vi "Teleop.vi"(10 "Match Info":T3={"Autonomous Elapsed Seconds"=0.0, "TeleOp Elapsed Seconds"=0.0, "Disabled Elapsed Seconds"=0.0, "Visited Autonomous"=FALSE, "Visited TeleOp"=FALSE, "Visited Disabled"=FALSE, "Autonomous Settings"={"Autonomous Style"=enum."Independent", "VI Refnum"=refnum}}, 11 "Call Context":T4) -> ()   [LabVIEW 2020]
doc: "This VI is called for each TeleOp packet received from the DS where the robot is not disabled. It is often used to read from the joysticks and update I/O or to update setpoints for timed control loops. It should complete and return within 20 milliseconds or it may miss DS packets."
uses:
  <vilib>/Rock Robotics/WPI/DriverStation/WPI_DriverStationDerivedRobotMode.ctl
  <vilib>/Rock Robotics/WPI/DriverStation/WPI_DriverStationMatch Info.ctl
  <vilib>/Rock Robotics/WPI/ThirdParty/Sensors/navX/_TypeDefs/FRIC_navX_DeviceNumbersTypeDef.ctl
  981LabViewComponents/2023 Robot Global Data.vi
  <vilib>/Rock Robotics/WPI/Utilities/WPI_GetSetVariantRefNum.vi
  <vilib>/Rock Robotics/Network Tables/NT Write Boolean Array.vi
  <vilib>/Rock Robotics/Network Tables/NT Write Numeric Array.vi
  <vilib>/Rock Robotics/Network Tables/NT Read Boolean.vi
  <vilib>/Rock Robotics/Network Tables/NT Read Number.vi
  <vilib>/Rock Robotics/Network Tables/NT Write Number.vi
panel:
  out "armSensor":dbl
  out "wristSensor":dbl
  out "armTarget":dbl
  out "wristTarget":dbl
  out "teleopState":T1(ring)
  out "displayTeleopCounter":i32
  out "Raw Values":T2 {"Accel X" format="%.8f"; "Accel Y" format="%.8f"; "Accel Z" format="%.8f"; "Gyro X" format="%.8f"; "Gyro Y" format="%.8f"; "Gyro Z" format="%.8f"; "Mag X" format="%.8f"; "Mag Y" format="%.8f"; "Mag Z" format="%.8f"}
  out "Sample Slider 0":dbl(slide) scale=0.0..5.0
  out "Sample Boolean 1":bool
  out "Sample Boolean 0":bool
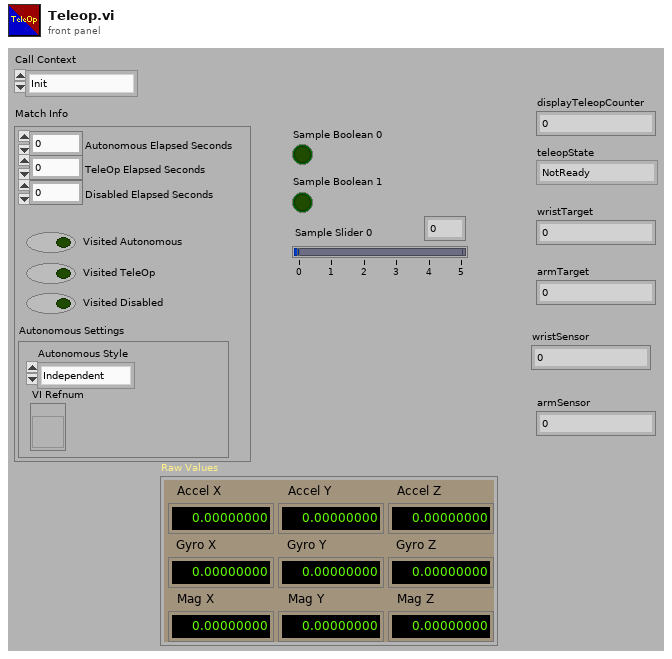
[diagram p1: front panel]
types:
  T1 = enum16{"NotReady", "Init", "UnstowA", "UnstowB", "UnstowC", "Teleop", "StowA", "StowB", "StowC"}
  T2 = cluster{"Accel X":dbl, "Accel Y":dbl, "Accel Z":dbl, "Gyro X":dbl, "Gyro Y":dbl, "Gyro Z":dbl, "Mag X":dbl, "Mag Y":dbl, "Mag Z":dbl}
  T3 = typedef "WPI_DriverStationMatch Info.ctl" = cluster{"Autonomous Elapsed Seconds":dbl, "TeleOp Elapsed Seconds":dbl, "Disabled Elapsed Seconds":dbl, "Visited Autonomous":bool, "Visited TeleOp":bool, "Visited Disabled":bool, "Autonomous Settings":cluster{"Autonomous Style":enum16{"Iterative", "Independent"}, "VI Refnum":refnum<vi>}}
  T4 = typedef "WPI_DriverStationDerivedRobotMode.ctl" = enum16{"Init", "Execute", "Stop"}
  T5 = typedef "WPI_JoystickDevRef.ctl" = cluster{"Device":T6}
  T6 = typedef "WPI_JoystickDeviceEnum.ctl" = enum16{"USB 0", "USB 1", "USB 2", "USB 3", "USB 4", "USB 5"}
  T7 = typedef "FRIC_navX_DeviceNumbersTypeDef.ctl" = enum16{"Dev0", "Dev1", "Dev2", "Dev3"}
  T8 = typedef "WPI_RobotDriveDevRef.ctl" = cluster{"DevStatus":errorcluster, "Motors[]":T9[], "Square Inputs":bool, "Max Output":dbl}
  T9 = typedef "WPI_MotorControlDeviceRef.ctl" = cluster{"DeviceStatus":errorcluster, "Type":T10, "PWM":cluster{"PWM Channel":T11, "DeadBand":T12}, "CAN":cluster{"Device Number":u8, "SetOutput VI Ref":variant, "GetOutput VI Ref":variant, "Enable VI Ref":variant, "Disable VI Ref":variant, "Data":variant}, "Invert":bool, "DIO PWM":cluster{"PWM \"Enable\" Channel":T11, "DIOChannel":T13, "PWM Rate":dbl}}
  T10 = typedef "WPI_MotorControlType.ctl" = enum16{"PWM", "CAN", "DIO PWM"}
  T11 = typedef "FPGA_DIOPWMChannel.ctl" = enum8{"PWM 0", "PWM 1", "PWM 2", "PWM 3", "PWM 4", "PWM 5", "PWM 6", "PWM 7", "PWM 8", "PWM 9", "PWM MXP 0", "PWM MXP 1", "PWM MXP 2", "PWM MXP 3", "PWM MXP 4", "PWM MXP 5", "PWM MXP 6", "PWM MXP 7", "PWM MXP 8", "PWM MXP 9", "Invalid"}
  T12 = typedef "WPI_PWMDeadband.ctl" = cluster{"Name":string, "maxPositivePwm":i32, "minPositivePwm":i32, "centerPwm":i32, "maxNegativePwm":i32, "minNegativePwm":i32, "angularRange":u16}
  T13 = typedef "FPGA_DIOChannel.ctl" = enum8{"DIO 0", "DIO 1", "DIO 2", "DIO 3", "DIO 4", "DIO 5", "DIO 6", "DIO 7", "DIO 8", "DIO 9", "DIO MXP 0", "DIO MXP 1", "DIO MXP 2", "DIO MXP 3", "DIO MXP 4", "DIO MXP 5", "DIO MXP 6", "DIO MXP 7", "DIO MXP 8", "DIO MXP 9", "DIO MXP 10", "DIO MXP 11", "DIO MXP 12", "DIO MXP 13", "DIO MXP 14", "DIO MXP 15", "SPI Port CS1", "SPI Port CS2", "SPI Port CS3", "SPI Port MISO", "SPI Port MOSI", "Invalid"}
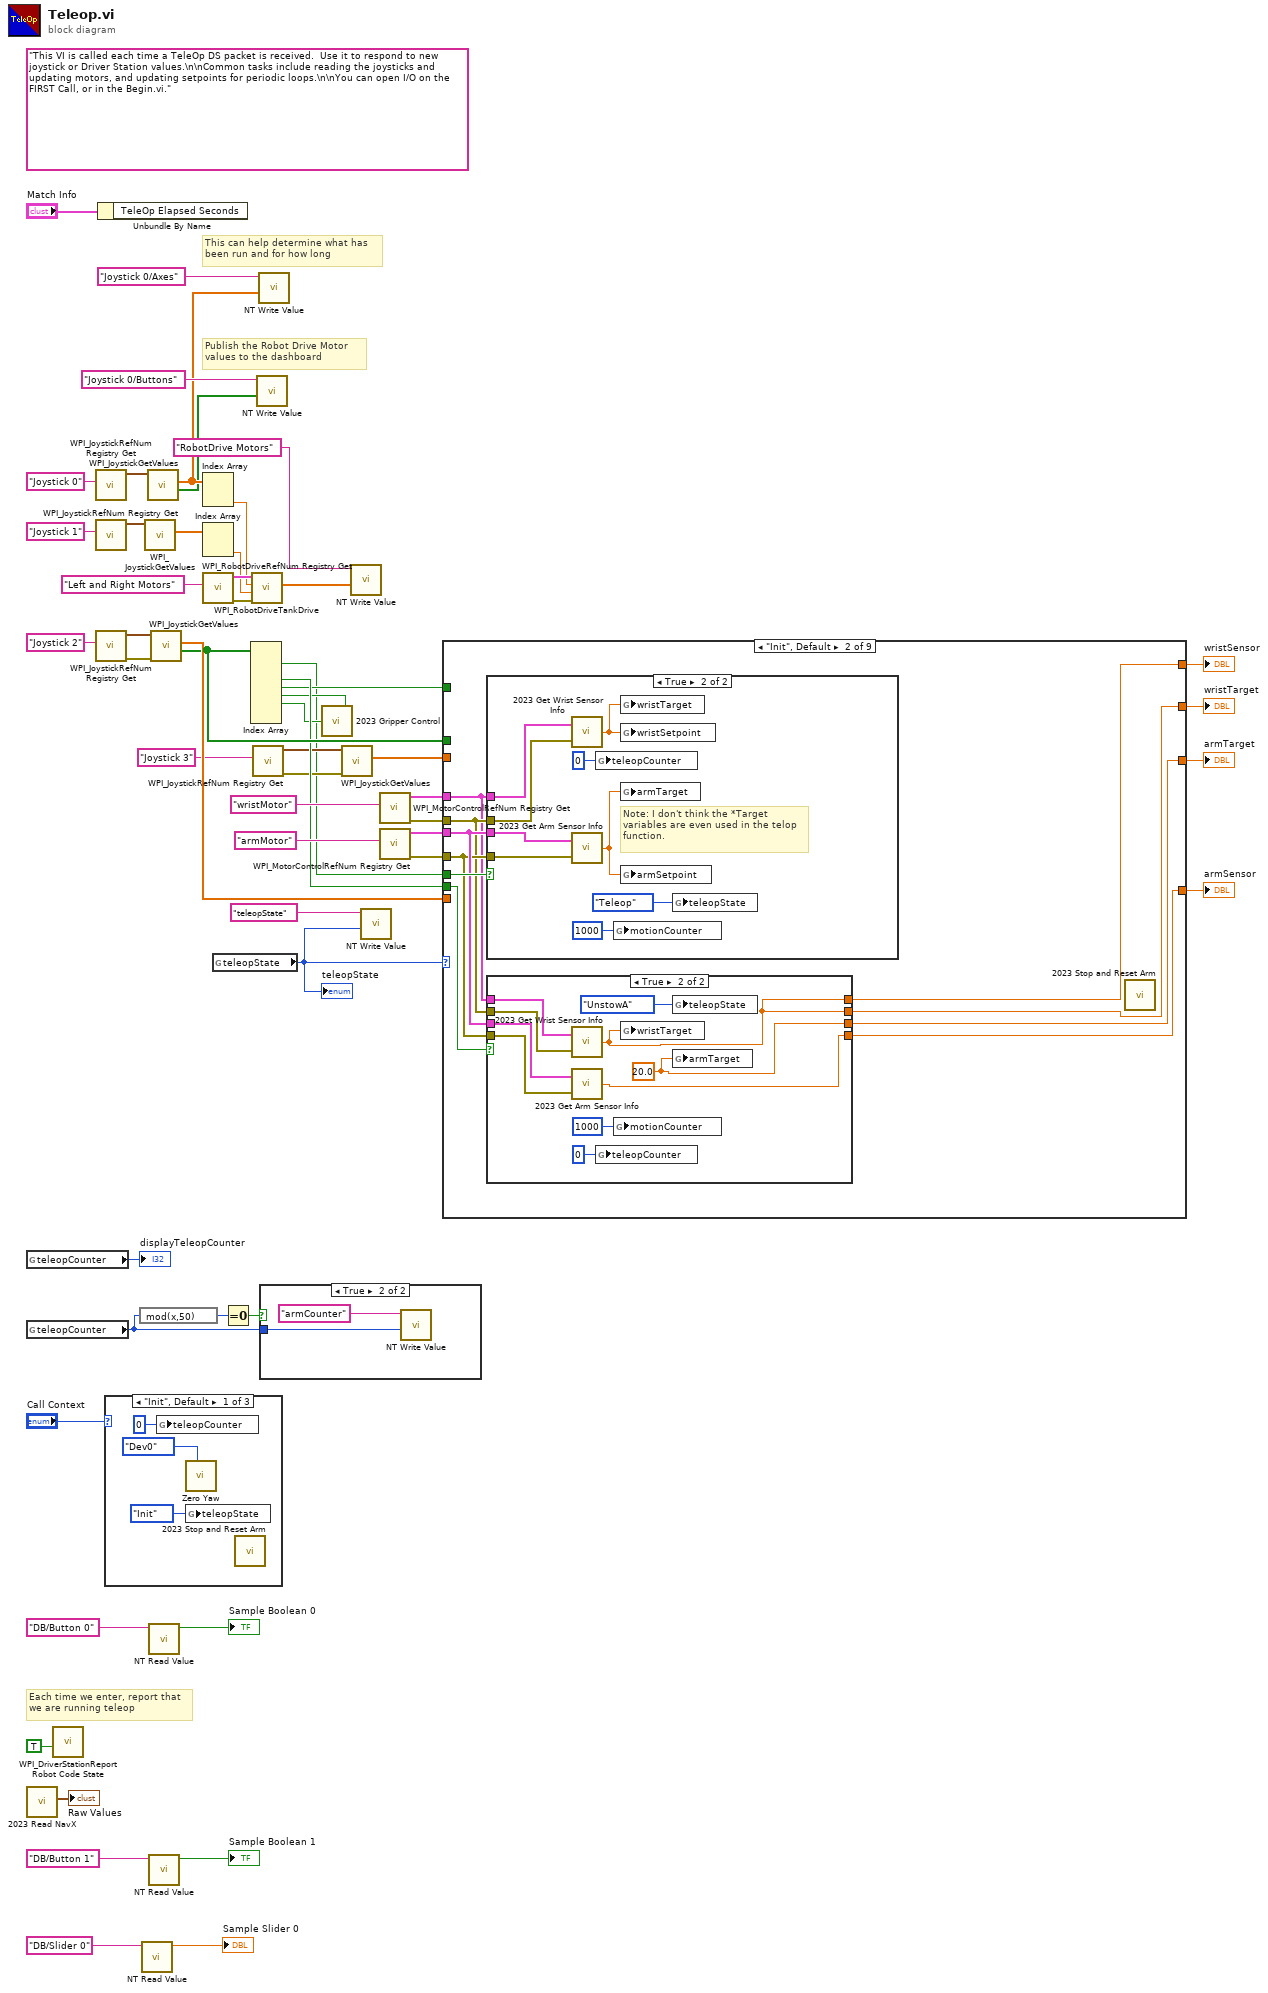
[diagram p0: block diagram]
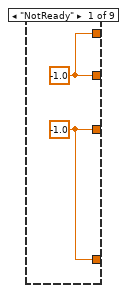
[diagram p2: hidden frame]
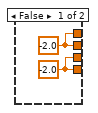
[diagram p4: hidden frame]
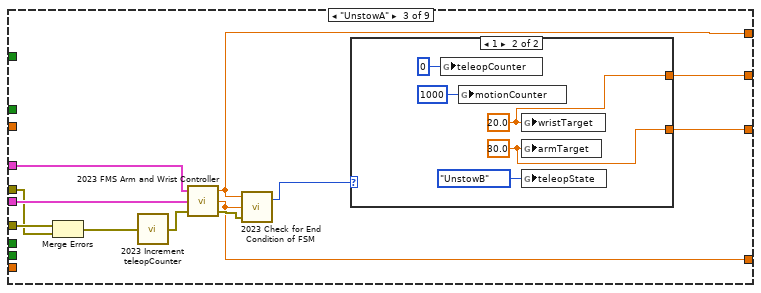
[diagram p5: hidden frame]
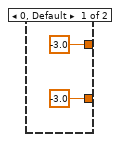
[diagram p6: hidden frame]
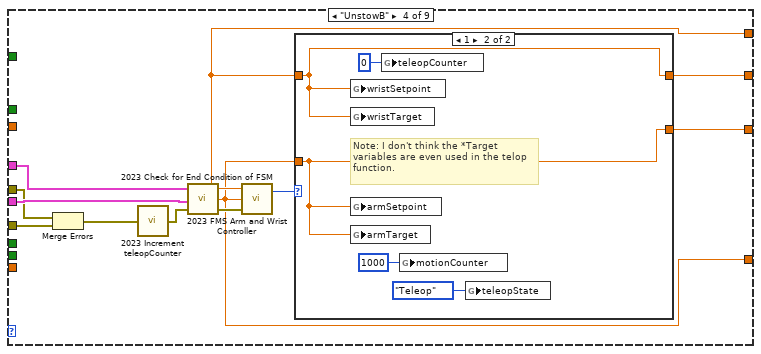
[diagram p7: hidden frame]
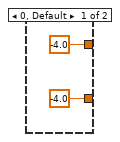
[diagram p8: hidden frame]
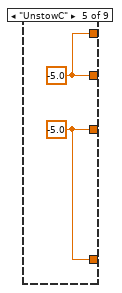
[diagram p9: hidden frame]
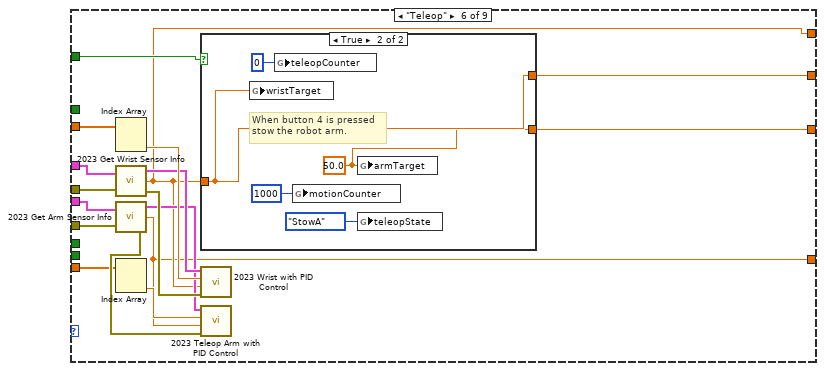
[diagram p10: hidden frame]
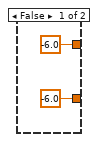
[diagram p11: hidden frame]
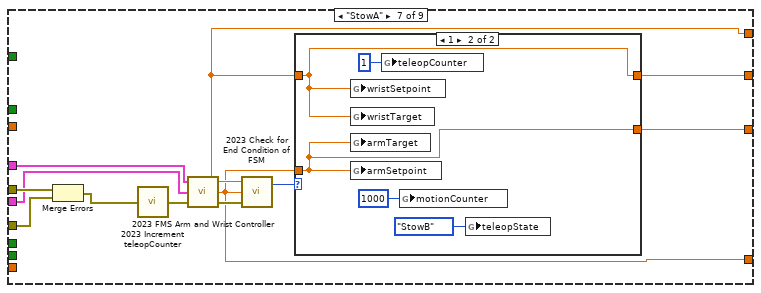
[diagram p12: hidden frame]
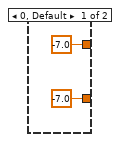
[diagram p13: hidden frame]
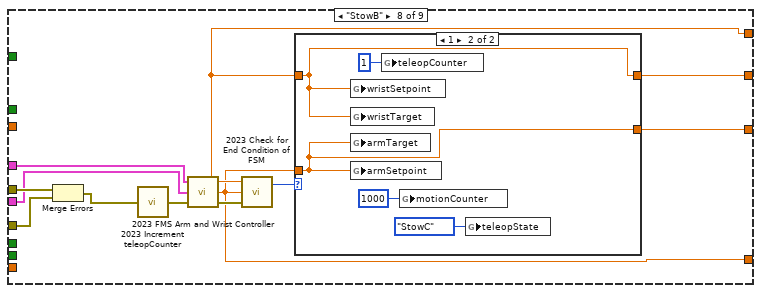
[diagram p14: hidden frame]
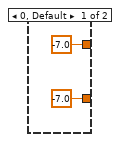
[diagram p15: hidden frame]
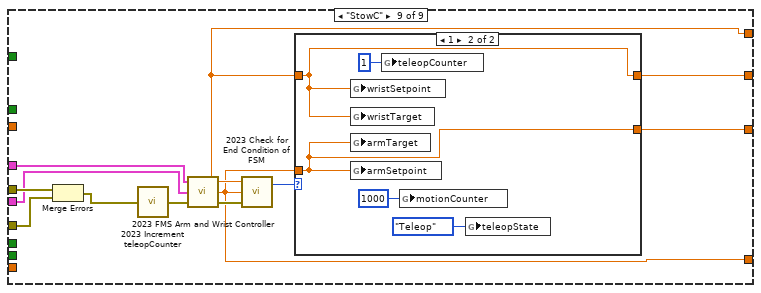
[diagram p16: hidden frame]
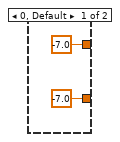
[diagram p17: hidden frame]
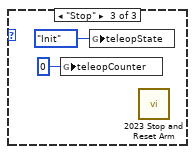
[diagram p20: hidden frame]
diagram:
  (unwired) "This VI is called each time a TeleOp DS packet is received.  Use it to respond to new joystick or Driver Station values.\n\nCommon tasks include reading the joysticks and updating motors, and updating setpoints for periodic loops.\n\nYou can open I/O on the FIRST Call, or in the Begin.vi."
  # "Publish the Robot Drive Motor\nvalues to the dashboard"
  # "Each time we enter, report that\nwe are running teleop"
  # "This can help determine what has\nbeen run and for how long"
  n1 = global read "2023 Robot Global Data.vi" "teleopCounter"() -> (→"displayTeleopCounter":i32)
  n2 = global read "2023 Robot Global Data.vi" "teleopCounter"() -> (w29:i32)
  n3 = call "2023 Read NavX.vi"() -> ("Raw Values"=→"Raw Values":T2)  [unwired: 4 out]
  n4 = call <vilib>:"WPI_DriverStationReport Robot Code State.vi"("TeleOp"=TRUE ("Autonomous")) -> ()  [unwired: 10 in, 1 out]
  n5 = call <vilib>:"WPI_JoystickRefNum Registry Get.vi"("refnum name"="Joystick 0") -> ("JoystickDevRef"=w53:T5)  [unwired: 1 in, 9 out]
  n6 = call <vilib>:"WPI_JoystickRefNum Registry Get.vi"("refnum name"="Joystick 1") -> ("JoystickDevRef"=w34:T5)  [unwired: 1 in, 9 out]
  n7 = call <vilib>:"WPI_JoystickRefNum Registry Get.vi"("refnum name"="Joystick 2") -> ("error out"=w21:errorcluster, "JoystickDevRef"=w23:T5)  [unwired: 1 in, 8 out]
  n8 = Unbundle By Name("Match Info") -> ()  [unwired: 1 out]
  n9 = case shown="\"Init\", Default" "Call Context" {
    frame "Init", Default {
      n10 = global write "2023 Robot Global Data.vi" "teleopCounter"(0 ("armCounter")) -> ()
      n11 = call <vilib>:"Zero Yaw.vi"("Device Number"=FRIC_navX_DeviceNumbersTypeDef."Dev0") -> ()  [unwired: 11 in]
      n12 = global write "2023 Robot Global Data.vi" "teleopState"(T1."Init" ("teleopState")) -> ()
      n13 = call "2023 Stop and Reset Arm.vi"() -> ()  [unwired: 1 in, 1 out]
    }
    frame "Execute" {
    }
    frame "Stop" {
      n14 = global write "2023 Robot Global Data.vi" "teleopCounter"(0 ("armCounter")) -> ()
      n15 = global write "2023 Robot Global Data.vi" "teleopState"(T1."Init" ("teleopState")) -> ()
      n16 = call "2023 Stop and Reset Arm.vi"() -> ()  [unwired: 1 in, 1 out]
    }
  }
  n17 = expression code="mod(x,50)"(w29) -> (w30:i32)
  n18 = call-poly <vilib>:"NT Read Value.vi"("name"="DB/Slider 0" ("refnum name")) -> ("value"=→"Sample Slider 0":dbl)  [unwired: 8 in, 2 out]
  n19 = call <vilib>:"WPI_JoystickGetValues.vi"("JoystickDevRef"=w34) -> ("Axes"=w33:dbl[])  [unwired: 6 in, 4 out]
  n20 = call <vilib>:"WPI_JoystickGetValues.vi"("JoystickDevRef"=w53) -> ("Buttons"=w48:bool[], "Axes"=w49:dbl[])  [unwired: 6 in, 3 out]
  n21 = call-poly <vilib>:"NT Read Value.vi"("name"="DB/Button 0" ("refnum name")) -> ("value"=→"Sample Boolean 0":bool)  [unwired: 8 in, 2 out]
  n22 = call-poly <vilib>:"NT Read Value.vi"("name"="DB/Button 1" ("refnum name")) -> ("value"=→"Sample Boolean 1":bool)  [unwired: 8 in, 2 out]
  n23 = call <vilib>:"WPI_JoystickGetValues.vi"("error in (no error)"=w21, "JoystickDevRef"=w23) -> ("Buttons"=w19:bool[], "Axes"=w20:dbl[])  [unwired: 5 in, 3 out]
  n24 = Index Array(array=w49) -> (element #2=w32:dbl)  [unwired: 2 in, 1 out]
  n25 = Index Array(array=w33) -> (element #2=w31:dbl)  [unwired: 2 in, 1 out]
  n26 = call <vilib>:"WPI_RobotDriveRefNum Registry Get.vi"("refnum name"="Left and Right Motors") -> ("error out"=w37:errorcluster, "RobotDriveDevRef"=w38:T8)  [unwired: 1 in, 8 out]
  n27 = global read "2023 Robot Global Data.vi" "teleopState"() -> (w1:T1)
  "teleopState" <- w1
  n28 = Equal To 0?(x=w30) -> (x = 0?=w28:bool)
  n29 = Index Array(array=w19) -> (element #1=w5:bool, element #3=w18:bool, element #4=w13:bool, element #5=w9:bool, element #6=w10:bool)  [unwired: 8 in, 3 out]
  n30 = call <vilib>:"WPI_RobotDriveTankDrive.vi"("error in (no error)"=w37, "Right axis value"=w31, "Left axis value"=w32, "RobotDriveDevRef"=w38) -> ("Motor Values"=w36:dbl[])  [unwired: 5 in, 2 out]
  n31 = call <vilib>:"WPI_JoystickRefNum Registry Get.vi"("refnum name"="Joystick 3") -> ("error out"=w15:errorcluster, "JoystickDevRef"=w16:T5)  [unwired: 1 in, 8 out]
  n32 = call-poly <vilib>:"NT Write Value.vi"("value"=w48, "name"="Joystick 0/Buttons" ("Name")) -> ()  [unwired: 9 in, 1 out]
  n33 = call-poly <vilib>:"NT Write Value.vi"("value"=w49, "name"="Joystick 0/Axes" ("Name")) -> ()  [unwired: 9 in, 1 out]
  n34 = case shown="True" w28 {
    tunnel: w29 -> [_ w62]
    frame False {
    }
    frame True {
      n35 = call-poly <vilib>:"NT Write Value.vi"("value"=w62, "name"="armCounter") -> ()  [unwired: 9 in, 1 out]
    }
  }
  n36 = call "2023 Gripper Control.vi"("Button 5"=w9, "Button 6"=w10) -> ()
  n37 = call <vilib>:"WPI_JoystickGetValues.vi"("error in (no error)"=w15, "JoystickDevRef"=w16) -> ("Axes"=w14:dbl[])  [unwired: 5 in, 4 out]
  n38 = call-poly <vilib>:"NT Write Value.vi"("value"=w36, "name"="RobotDrive Motors" ("Name")) -> ()  [unwired: 9 in, 1 out]
  n39 = call-poly <vilib>:"NT Write Value.vi"("value"=w1, "name"="teleopState") -> ()  [unwired: 9 in, 1 out]
  n40 = call <vilib>:"WPI_MotorControlRefNum Registry Get.vi"("refnum name"="wristMotor") -> ("error out"=w12:errorcluster, "MotorControlDevRef"=w24:T9)  [unwired: 9 in]
  n41 = call <vilib>:"WPI_MotorControlRefNum Registry Get.vi"("refnum name"="armMotor") -> ("error out"=w11:errorcluster, "MotorControlDevRef"=w25:T9)  [unwired: 9 in]
  n42 = case shown="\"Init\", Default" w1 {
    tunnel: w25 -> [_ w69 w107 w126 _ w143 w167 w186 w205]
    tunnel: w24 -> [_ w66 w108 w127 _ w149 w168 w187 w206]
    tunnel: w20 -> [_ _ _ _ _ w148 _ _ _]
    tunnel: w19 -> [_ _ _ _ _ _ _ _ _]
    tunnel: w18 -> [_ w75 _ _ _ _ _ _ _]
    tunnel: w14 -> [_ _ _ _ _ w147 _ _ _]
    tunnel: w13 -> [_ _ _ _ _ w146 _ _ _]
    tunnel: w12 -> [_ w67 w105 w124 _ w144 w172 w191 w210]
    tunnel: w11 -> [_ w68 w106 w125 _ w145 w171 w190 w209]
    tunnel: [w65 w74 w100 w119 w136 w140 w164 w183 w202] -> w7
    tunnel: [w64 w73 w99 w118 w135 w139 w163 w182 w201] -> w6
    tunnel: w5 -> [_ w72 _ _ _ _ _ _ _]
    tunnel: [w65 w70 w98 w117 w136 w138 w162 w181 w200] -> w4
    tunnel: [w64 w71 w97 w116 w135 w137 w161 w180 w199] -> w3
    frame "NotReady" {
      w64 = -1.0 ("armSensorPosition")
      w65 = -1.0 ("wristSensorPosition")
    }
    frame "Init", Default {
      n43 = case shown="True" w72 {
        tunnel: w69 -> [_ w81]
        tunnel: w68 -> [_ w80]
        tunnel: w66 -> [_ w79]
        tunnel: w67 -> [_ w78]
        frame False {
        }
        frame True {
          # "Note: I don't think the *Target\nvariables are even used in the telop\nfunction."
          n44 = call "2023 Get Wrist Sensor Info.vi"("MotorControlDevRefIn"=w79, "error in"=w78) -> ("wristSensorPosition"=w76:dbl)  [unwired: 2 out]
          n45 = call "2023 Get Arm Sensor Info.vi"("MotorControlDevRefIn"=w81, "error in (no error)"=w80) -> ("armSensorPosition"=w77:dbl)  [unwired: 2 out]
          n46 = global write "2023 Robot Global Data.vi" "teleopCounter"(0 ("armCounter")) -> ()
          n47 = global write "2023 Robot Global Data.vi" "motionCounter"(1000 ("motionCounter")) -> ()
          n48 = global write "2023 Robot Global Data.vi" "wristTarget"(w76) -> ()
          n49 = global write "2023 Robot Global Data.vi" "wristSetpoint"(w76) -> ()
          n50 = global write "2023 Robot Global Data.vi" "armTarget"(w77) -> ()
          n51 = global write "2023 Robot Global Data.vi" "armSetpoint"(w77) -> ()
          n52 = global write "2023 Robot Global Data.vi" "teleopState"(T1."Teleop" ("teleopState")) -> ()
        }
      }
      n53 = case shown="True" w75 {
        tunnel: w69 -> [_ w94]
        tunnel: w66 -> [_ w93]
        tunnel: w68 -> [_ w92]
        tunnel: w67 -> [_ w91]
        tunnel: [w86 w87] -> w74
        tunnel: [w85 w89] -> w73
        tunnel: [w85 w88] -> w71
        tunnel: [w86 w87] -> w70
        frame False {
          w85 = -2.0 ("armSensorPosition")
          w86 = -2.0 ("wristSensorPosition")
        }
        frame True {
          w89 = 20.0 ("armTarget")
          n54 = call "2023 Get Wrist Sensor Info.vi"("MotorControlDevRefIn"=w93, "error in"=w91) -> ("wristSensorPosition"=w87:dbl)  [unwired: 2 out]
          n55 = call "2023 Get Arm Sensor Info.vi"("MotorControlDevRefIn"=w94, "error in (no error)"=w92) -> ("armSensorPosition"=w88:dbl)  [unwired: 2 out]
          n56 = global write "2023 Robot Global Data.vi" "teleopCounter"(0 ("teleopCounter")) -> ()
          n57 = global write "2023 Robot Global Data.vi" "motionCounter"(1000 ("motionCounter")) -> ()
          n58 = global write "2023 Robot Global Data.vi" "wristTarget"(w87) -> ()
          n59 = global write "2023 Robot Global Data.vi" "teleopState"(T1."UnstowA" ("teleopState")) -> ()
          n60 = global write "2023 Robot Global Data.vi" "armTarget"(w89) -> ()
        }
      }
      n61 = call "2023 Stop and Reset Arm.vi"() -> ()  [unwired: 1 in, 1 out]
    }
    frame "UnstowA" {
      n62 = Merge Errors(w106, w105) -> (w101:errorcluster)
      n63 = call "2023 Increment teleopCounter.vi"("error in"=w101) -> ("error out"=w102:errorcluster)
      n64 = call "2023 FMS Arm and Wrist Controller.vi"("error in"=w102, "armMotorControlDevRef"=w107, "wristMotorControlDevRef"=w108) -> ("error out"=w104:errorcluster, "armSensorPosition"=w97:dbl, "wristSensorPosition"=w98:dbl)
      n65 = call "2023 Check for End Condition of FSM.vi"("error in"=w104, "armSensorPosition"=w97, "wristSensorPosition"=w98) -> ("timeToTransition"=w103:i32)  [unwired: 1 out]
      n66 = case shown="1" w103 {
        tunnel: [-3.0 ("wristSensorPosition") w112] -> w100
        tunnel: [-3.0 ("armSensorPosition") w111] -> w99
        frame 0, Default {
        }
        frame 1 {
          w111 = 30.0 ("armTarget")
          w112 = 20.0 ("wristTarget")
          n67 = global write "2023 Robot Global Data.vi" "teleopCounter"(0 ("armCounter")) -> ()
          n68 = global write "2023 Robot Global Data.vi" "motionCounter"(1000 ("motionCounter")) -> ()
          n69 = global write "2023 Robot Global Data.vi" "wristTarget"(w112) -> ()
          n70 = global write "2023 Robot Global Data.vi" "armTarget"(w111) -> ()
          n71 = global write "2023 Robot Global Data.vi" "teleopState"(T1."UnstowB" ("teleopState")) -> ()
        }
      }
    }
    frame "UnstowB" {
      n72 = Merge Errors(w124, w125) -> (w121:errorcluster)
      n73 = call "2023 Increment teleopCounter.vi"("error in"=w121) -> ("error out"=w120:errorcluster)
      n74 = call "2023 FMS Arm and Wrist Controller.vi"("error in"=w120, "armMotorControlDevRef"=w126, "wristMotorControlDevRef"=w127) -> ("error out"=w122:errorcluster, "armSensorPosition"=w116:dbl, "wristSensorPosition"=w117:dbl)
      n75 = call "2023 Check for End Condition of FSM.vi"("error in"=w122, "armSensorPosition"=w116, "wristSensorPosition"=w117) -> ("timeToTransition"=w123:i32)  [unwired: 1 out]
      n76 = case shown="1" w123 {
        tunnel: w117 -> [_ w131]
        tunnel: w116 -> [_ w130]
        tunnel: [-4.0 ("wristSensorPosition") w131] -> w119
        tunnel: [-4.0 ("armSensorPosition") w130] -> w118
        frame 0, Default {
        }
        frame 1 {
          # "Note: I don't think the *Target\nvariables are even used in the telop\nfunction."
          n77 = global write "2023 Robot Global Data.vi" "wristSetpoint"(w131) -> ()
          n78 = global write "2023 Robot Global Data.vi" "wristTarget"(w131) -> ()
          n79 = global write "2023 Robot Global Data.vi" "armSetpoint"(w130) -> ()
          n80 = global write "2023 Robot Global Data.vi" "armTarget"(w130) -> ()
          n81 = global write "2023 Robot Global Data.vi" "teleopCounter"(0 ("armCounter")) -> ()
          n82 = global write "2023 Robot Global Data.vi" "motionCounter"(1000 ("motionCounter")) -> ()
          n83 = global write "2023 Robot Global Data.vi" "teleopState"(T1."Teleop" ("teleopState")) -> ()
        }
      }
    }
    frame "UnstowC" {
      w135 = -5.0 ("armSensorPosition")
      w136 = -5.0 ("wristSensorPosition")
    }
    frame "Teleop" {
      n84 = Index Array(array=w147) -> (element #2=w152:dbl)  [unwired: 2 in, 1 out]
      n85 = call "2023 Get Wrist Sensor Info.vi"("MotorControlDevRefIn"=w149, "error in"=w144) -> ("MotorControlDevRefOut"=w142:T9, "wristSensorPosition"=w138:dbl, "error out"=w150:errorcluster)
      n86 = call "2023 Get Arm Sensor Info.vi"("MotorControlDevRefIn"=w143, "error in (no error)"=w145) -> ("MotorControlDevRefOut"=w141:T9, "armSensorPosition"=w137:dbl, "error out"=w151:errorcluster)
      n87 = Index Array(array=w148) -> (element #2=w153:dbl)  [unwired: 2 in, 1 out]
      n88 = case shown="True" w146 {
        tunnel: w138 -> [_ w157]
        tunnel: [-6.0 ("wristSensorPosition") w157] -> w140
        tunnel: [-6.0 ("armSensorPosition") w156] -> w139
        frame False {
        }
        frame True {
          w156 = 50.0 ("armTarget")
          # "When button 4 is pressed\nstow the robot arm."
          n89 = global write "2023 Robot Global Data.vi" "wristTarget"(w157) -> ()
          n90 = global write "2023 Robot Global Data.vi" "teleopCounter"(0 ("armCounter")) -> ()
          n91 = global write "2023 Robot Global Data.vi" "motionCounter"(1000 ("motionCounter")) -> ()
          n92 = global write "2023 Robot Global Data.vi" "armTarget"(w156) -> ()
          n93 = global write "2023 Robot Global Data.vi" "teleopState"(T1."StowA" ("teleopState")) -> ()
        }
      }
      n94 = call "2023 Wrist with PID Control.vi"("error in (no error)"=w150, "newWristSensorPosition"=w138, "Joystick Command"=w152, "MotorControlDevRef"=w142) -> ()  [unwired: 3 out]
      n95 = call "2023 Teleop Arm with PID Control.vi"("error in (no error)"=w151, "newArmSensorPosition"=w137, "Joystick Command"=w153, "MotorControlDevRef"=w141) -> ()  [unwired: 4 out]
    }
    frame "StowA" {
      n96 = Merge Errors(w172, w171) -> (w170:errorcluster)
      n97 = call "2023 Increment teleopCounter.vi"("error in"=w170) -> ("error out"=w166:errorcluster)
      n98 = call "2023 FMS Arm and Wrist Controller.vi"("error in"=w166, "armMotorControlDevRef"=w167, "wristMotorControlDevRef"=w168) -> ("error out"=w169:errorcluster, "armSensorPosition"=w161:dbl, "wristSensorPosition"=w162:dbl)
      n99 = call "2023 Check for End Condition of FSM.vi"("error in"=w169, "armSensorPosition"=w161, "wristSensorPosition"=w162) -> ("timeToTransition"=w165:i32)  [unwired: 1 out]
      n100 = case shown="1" w165 {
        tunnel: w162 -> [_ w176]
        tunnel: w161 -> [_ w175]
        tunnel: [-7.0 ("wristSensorPosition") w176] -> w164
        tunnel: [-7.0 ("armSensorPosition") w175] -> w163
        frame 0, Default {
        }
        frame 1 {
          n101 = global write "2023 Robot Global Data.vi" "wristSetpoint"(w176) -> ()
          n102 = global write "2023 Robot Global Data.vi" "wristTarget"(w176) -> ()
          n103 = global write "2023 Robot Global Data.vi" "armTarget"(w175) -> ()
          n104 = global write "2023 Robot Global Data.vi" "armSetpoint"(w175) -> ()
          n105 = global write "2023 Robot Global Data.vi" "teleopCounter"(1 ("armCounter")) -> ()
          n106 = global write "2023 Robot Global Data.vi" "motionCounter"(1000 ("motionCounter")) -> ()
          n107 = global write "2023 Robot Global Data.vi" "teleopState"(T1."StowB" ("teleopState")) -> ()
        }
      }
    }
    frame "StowB" {
      n108 = Merge Errors(w191, w190) -> (w189:errorcluster)
      n109 = call "2023 Increment teleopCounter.vi"("error in"=w189) -> ("error out"=w185:errorcluster)
      n110 = call "2023 FMS Arm and Wrist Controller.vi"("error in"=w185, "armMotorControlDevRef"=w186, "wristMotorControlDevRef"=w187) -> ("error out"=w188:errorcluster, "armSensorPosition"=w180:dbl, "wristSensorPosition"=w181:dbl)
      n111 = call "2023 Check for End Condition of FSM.vi"("error in"=w188, "armSensorPosition"=w180, "wristSensorPosition"=w181) -> ("timeToTransition"=w184:i32)  [unwired: 1 out]
      n112 = case shown="1" w184 {
        tunnel: w181 -> [_ w195]
        tunnel: w180 -> [_ w194]
        tunnel: [-7.0 ("wristSensorPosition") w195] -> w183
        tunnel: [-7.0 ("armSensorPosition") w194] -> w182
        frame 0, Default {
        }
        frame 1 {
          n113 = global write "2023 Robot Global Data.vi" "wristSetpoint"(w195) -> ()
          n114 = global write "2023 Robot Global Data.vi" "wristTarget"(w195) -> ()
          n115 = global write "2023 Robot Global Data.vi" "armTarget"(w194) -> ()
          n116 = global write "2023 Robot Global Data.vi" "armSetpoint"(w194) -> ()
          n117 = global write "2023 Robot Global Data.vi" "teleopCounter"(1 ("armCounter")) -> ()
          n118 = global write "2023 Robot Global Data.vi" "motionCounter"(1000 ("motionCounter")) -> ()
          n119 = global write "2023 Robot Global Data.vi" "teleopState"(T1."StowC" ("teleopState")) -> ()
        }
      }
    }
    frame "StowC" {
      n120 = Merge Errors(w210, w209) -> (w208:errorcluster)
      n121 = call "2023 Increment teleopCounter.vi"("error in"=w208) -> ("error out"=w204:errorcluster)
      n122 = call "2023 FMS Arm and Wrist Controller.vi"("error in"=w204, "armMotorControlDevRef"=w205, "wristMotorControlDevRef"=w206) -> ("error out"=w207:errorcluster, "armSensorPosition"=w199:dbl, "wristSensorPosition"=w200:dbl)
      n123 = call "2023 Check for End Condition of FSM.vi"("error in"=w207, "armSensorPosition"=w199, "wristSensorPosition"=w200) -> ("timeToTransition"=w203:i32)  [unwired: 1 out]
      n124 = case shown="1" w203 {
        tunnel: w200 -> [_ w214]
        tunnel: w199 -> [_ w213]
        tunnel: [-7.0 ("wristSensorPosition") w214] -> w202
        tunnel: [-7.0 ("armSensorPosition") w213] -> w201
        frame 0, Default {
        }
        frame 1 {
          n125 = global write "2023 Robot Global Data.vi" "wristSetpoint"(w214) -> ()
          n126 = global write "2023 Robot Global Data.vi" "wristTarget"(w214) -> ()
          n127 = global write "2023 Robot Global Data.vi" "armTarget"(w213) -> ()
          n128 = global write "2023 Robot Global Data.vi" "armSetpoint"(w213) -> ()
          n129 = global write "2023 Robot Global Data.vi" "teleopCounter"(1 ("armCounter")) -> ()
          n130 = global write "2023 Robot Global Data.vi" "motionCounter"(1000 ("motionCounter")) -> ()
          n131 = global write "2023 Robot Global Data.vi" "teleopState"(T1."Teleop" ("teleopState")) -> ()
        }
      }
    }
  }
  "wristTarget" <- w7
  "armTarget" <- w6
  "wristSensor" <- w4
  "armSensor" <- w3
